vi "getUserEvent.vi"(8 "error in (no error)":errorcluster, 11 "GeneralDisplay in":refnum<class "GeneralDisplay.lvclass">) -> (0 "error out":errorcluster, 2 "UserEvent":refnum<user-event>, 3 "GeneralDisplay out":refnum<class "GeneralDisplay.lvclass">)   [LabVIEW 2018, in "GeneralDisplay.lvclass"]
uses:
  GeneralDisplay.lvclass
  Observer/Observer.lvclass
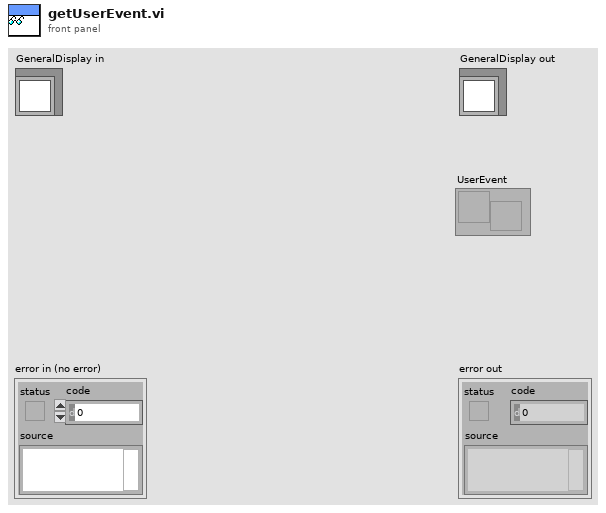
[diagram p1: front panel]
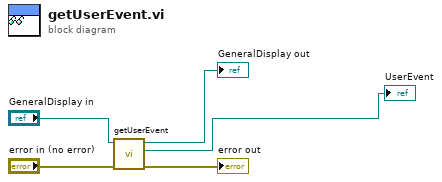
[diagram p0: block diagram]
diagram:
  n1 = call-parent "getUserEvent.vi"("error in (no error)"="error in (no error)", "Observer in"="GeneralDisplay in") -> ("error out"=→"error out":errorcluster, "UserEvent"=→"UserEvent":refnum<user-event>, "Observer out"=→"GeneralDisplay out":refnum<class "GeneralDisplay.lvclass">)  [unwired: 7 in]
